vi "Shooter Tilter Auto Manual.vi"(8 "changeMode":bool, 11 "joystickNumber":dbl) -> ()   [LabVIEW 2012]
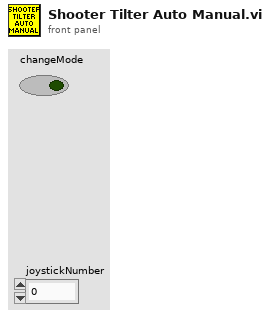
[diagram p1: front panel]
types:
  T1 = typedef "WPI_MotorControlDeviceRef.ctl" = cluster{"DeviceStatus":errorcluster, "Type":enum16{"PWM", "CAN"}, "PWM":cluster{"Digital Module":T2, "PWM Channel":T3, "DeadBand":T4}, "CAN":cluster{"Device Number":u8, "Control Mode":T5, "Semaphore":T6, "Max Vout":dbl}, "Invert":bool, "TransformRef":T7, "InvTransformRef":T7}
  T2 = typedef "FPGA_TypedefDigitalModule.ctl" = enum16{"Digital Module 1", "Digital Module 2"}
  T3 = typedef "FPGA_DIOPWMChannel.ctl" = enum8{"PWM 1", "PWM 2", "PWM 3", "PWM 4", "PWM 5", "PWM 6", "PWM 7", "PWM 8", "PWM 9", "PWM 10", "Invalid"}
  T4 = typedef "WPI_PWMDeadband.ctl" = cluster{"Name":string, "maxPositivePwm":i32, "minPositivePwm":i32, "centerPwm":i32, "maxNegativePwm":i32, "minNegativePwm":i32, "angularRange":u16}
  T5 = typedef "WPI_CANJaguar_ControlMode.ctl" = enum8{"Percent VBus", "Current", "Speed", "Position", "Voltage"}
  T6 = typedef "Semaphore RefNum" = refnum<k1>
  T7 = typedef "WPI_PWMTransform_ConPane.ctl" = refnum<vi>
  T8 = typedef "WPI_AnalogChannelDevRef.ctl" = cluster{"DevStatus":errorcluster, "Analog Module":T9, "Analog Channel":T10}
  T9 = typedef "FPGA_TypedefAnalogModule.ctl" = enum16{"Analog Module 1", "Analog Module 2"}
  T10 = typedef "FPGA_AIChannel.ctl" = enum8{"AI 1", "AI 2", "AI 3", "AI 4", "AI 5", "AI 6", "AI 7", "AI 8", "Invalid"}
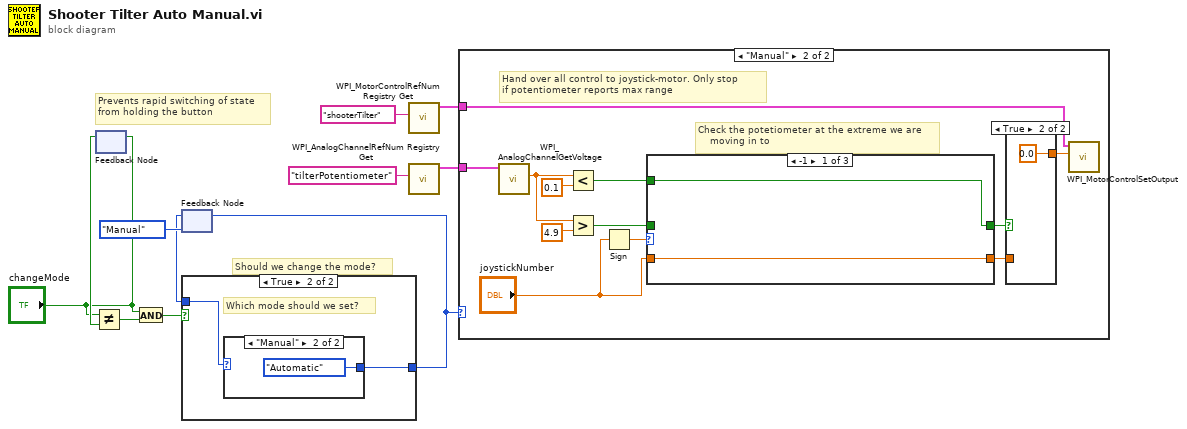
[diagram p0: block diagram]
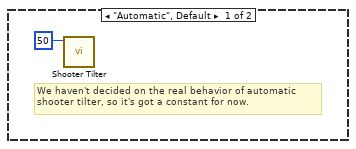
[diagram p2: hidden frame]
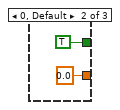
[diagram p4: hidden frame]
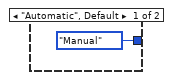
[diagram p7: hidden frame]
diagram:
  # "Prevents rapid switching of state\nfrom holding the button"
  # "Should we change the mode?"
  n1 = feedback-in #1("changeMode") -> ()
  n2 = feedback #1() -> (w2:bool)  [unwired: 1 in]
  n3 = Not Equal?(x="changeMode", y=w2) -> (x != y?=w3:bool)
  n4 = And(x="changeMode", y=w3) -> (x .and. y?=w4:bool)
  n5 = feedback #2(enum16{"Automatic", "Manual"}."Manual") -> (w10:enum16{"Automatic", "Manual"})
  n6 = case shown="True" w4 {
    tunnel: w10 -> [w12 w14]
    tunnel: [w12 w13] -> w9
    frame False {
    }
    frame True {
      # "Which mode should we set?"
      n7 = case shown="\"Manual\"" w14 {
        tunnel: [enum16{"Automatic", "Manual"}."Manual" enum16{"Automatic", "Manual"}."Automatic"] -> w13
        frame "Automatic", Default {
        }
        frame "Manual" {
        }
      }
    }
  }
  n8 = feedback-in #2(w9) -> ()
  n9 = call <vilib>:"WPI_MotorControlRefNum Registry Get.vi"("refnum name"="shooterTilter") -> ("MotorControlDevRef"=w5:T1)  [unwired: 9 in, 1 out]
  n10 = call <vilib>:"WPI_AnalogChannelRefNum Registry Get.vi"("refnum name"="tilterPotentiometer") -> ("AIDeviceRef"=w6:T8)  [unwired: 9 in, 1 out]
  n11 = case shown="\"Manual\"" w9 {
    tunnel: w6 -> [_ w29]
    tunnel: w5 -> [_ w25]
    frame "Automatic", Default {
      # "We haven't decided on the real behavior of automatic\nshooter tilter, so it's got a constant for now."
      n12 = call "Shooter Tilter.vi"("numericInput"=50) -> ()  [unwired: 11 in]
    }
    frame "Manual" {
      # "Check the potetiometer at the extreme we are\n    moving in to"
      # "Hand over all control to joystick-motor. Only stop\nif potentiometer reports max range"
      n13 = call <vilib>:"WPI_AnalogChannelGetVoltage.vi"("AIDeviceRef"=w29) -> ("Voltage"=w27:dbl)  [unwired: 8 in, 2 out]
      n14 = Less?(x=w27, y=0.1) -> (x < y?=w23:bool)
      n15 = Greater?(x=w27, y=4.9) -> (0:w22:bool)
      n16 = Sign(1:"joystickNumber") -> (0:w24:dbl)
      n17 = case shown="-1" w24 {
        tunnel: w23 -> [w33 _ _]
        tunnel: w22 -> [_ _ w37]
        tunnel: [w33 TRUE w37] -> w20
        tunnel: "joystickNumber" -> [w32 _ w36]
        tunnel: [w32 0.0 ("joystickNumber") w36] -> w19
        frame -1 {
        }
        frame 0, Default {
        }
        frame 1 {
        }
      }
      n18 = case shown="True" w20 {
        tunnel: w19 -> [w30 _]
        tunnel: [w30 0.0 ("joystickNumber")] -> w18
        frame False {
        }
        frame True {
        }
      }
      n19 = call <vilib>:"WPI_MotorControlSetOutput.vi"("Output"=w18, "MotorControlDevRef"=w25) -> ()  [unwired: 7 in, 3 out]
    }
  }
